vi "DAQ_SampleLoopSub.vi"(0 "DAQ_collectQueue":refnum<queue>, 1 "SampleSettings":T1={"samples per channel"=100, "SampleRate"=1000.0, "TansMaxLength"=500000.0, "ReadTimeOut"=10.0, "时钟源"=""}, 2 "AI_task":refnum<k21> caption="AITask", 3 "CntTask 1":refnum<k21> caption="CntTask1", 4 "CntTask 2":refnum<k21> caption="CntTask2", 6 "ClearCnt":bool, 8 "sensor_arrtribute":cluster{"Scale":dbl, "Offset":dbl}[](array[cluster])) -> (15 "RealTimeValue":dbl[](array[numeric]))   [LabVIEW 2020, in "DAQ.lvlib" / "NI_DAQ.lvclass"]
uses:
  NI_DAQ.lvclass
  DAQ_Base_class/protected/SampleSettings.ctl
  <vilib>/DAQmx/read.llb/DAQmx Read (Counter 1D DBL 1Chan NSamp).vi
  <vilib>/DAQmx/read.llb/DAQmx Read (Analog 2D DBL NChan NSamp).vi
  <vilib>/DAQmx/miscellaneous.llb/DAQmx Fill In Error Info.vi
  DAQ_Base_class/DAQ_Base.lvclass
panel:
  out "error out":errorcluster
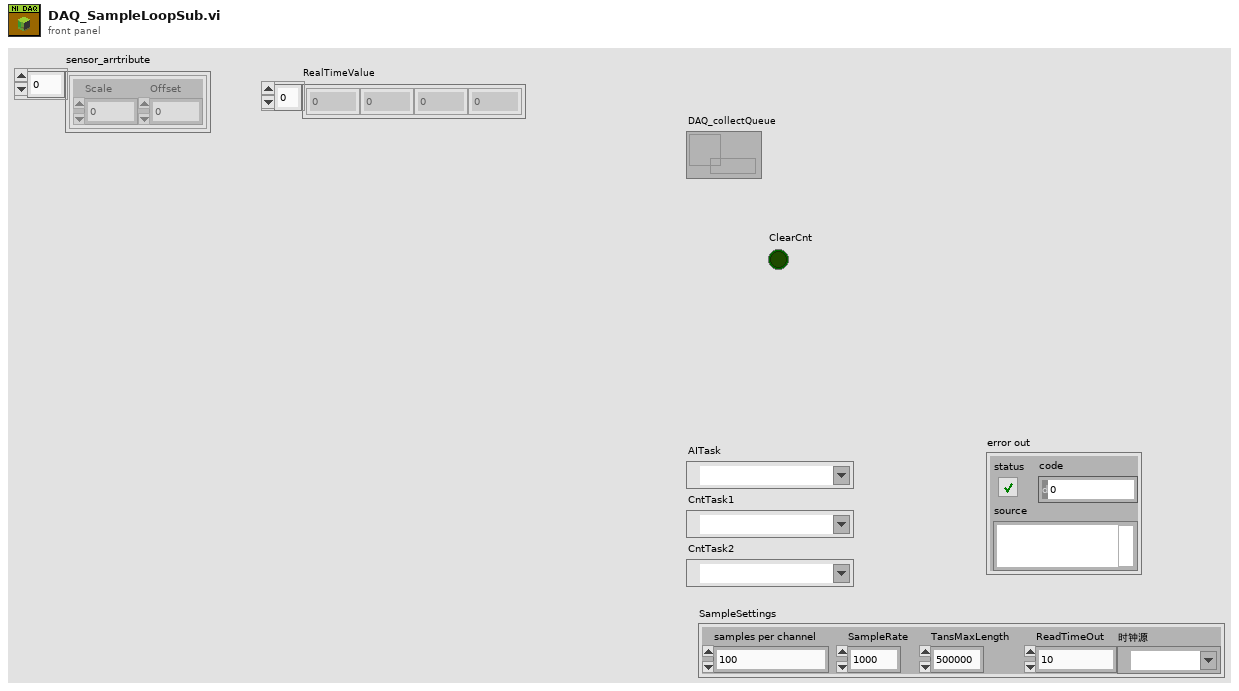
[diagram p1: front panel]
types:
  T1 = typedef "DAQ.lvlib/DAQ_Base.lvclass/SampleSettings.ctl" = cluster{"samples per channel":i32, "SampleRate":dbl, "TansMaxLength":dbl, "ReadTimeOut":dbl, "时钟源":tag}
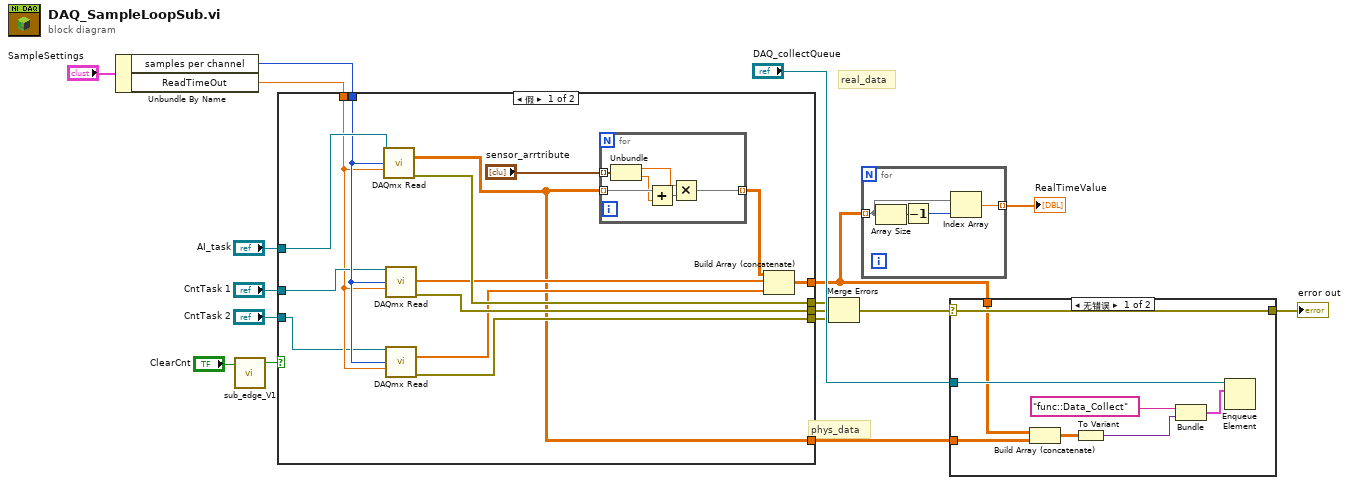
[diagram p0: block diagram]
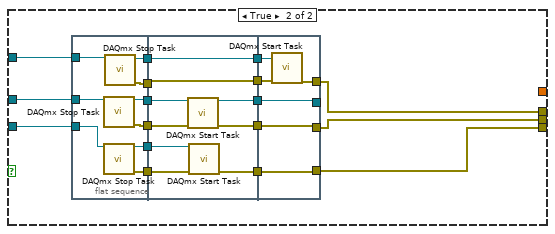
[diagram p2: hidden frame]
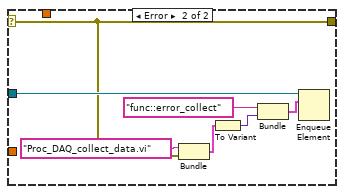
[diagram p3: hidden frame]
diagram:
  # "phys_data"
  # "real_data"
  n1 = Unbundle By Name("SampleSettings") -> ("samples per channel"=w9:i32, "ReadTimeOut"=w3:dbl)
  n2 = call "sub_edge_V1.vi"("signal_in"="ClearCnt") -> ("raise_edge"=w7:bool)  [unwired: 8 in, 2 out]
  n3 = case shown="假" w7 {
    tunnel: [w31 w46] -> w15
    tunnel: [w30 w45] -> w14
    tunnel: [w29 w44] -> w13
    tunnel: "AI_task" -> [w26 w43]
    tunnel: w9 -> [w25 _]
    tunnel: "CntTask 1" -> [w24 w42]
    tunnel: "CntTask 2" -> [w22 w41]
    tunnel: [w18 _] -> w1
    tunnel: [w20 _] -> w4
    tunnel: w3 -> [w23 _]
    frame False {
      n4 = call-poly <vilib>:"DAQmx Read.vi"("task/channels in"=w26, "number of samples per channel"=w25, "timeout"=w23) -> ("data"=w20:dbl[][], "error out"=w31:errorcluster)  [unwired: 10 in, 1 out]
      n5 = call-poly <vilib>:"DAQmx Read.vi"("task/channels in"=w24, "number of samples per channel"=w25, "timeout"=w23) -> ("data"=w27:dbl[], "error out"=w30:errorcluster)  [unwired: 10 in, 1 out]
      n6 = call-poly <vilib>:"DAQmx Read.vi"("task/channels in"=w22, "number of samples per channel"=w25, "timeout"=w23) -> ("data"=w28:dbl[], "error out"=w29:errorcluster)  [unwired: 10 in, 1 out]
      n7 = for {
        tunnel: w20 -> [w36] mode=indexing
        tunnel: "sensor_arrtribute" -> [w37] mode=indexing
        tunnel: [w32] -> w19 mode=indexing
        n8 = Unbundle(w37) -> ("Scale"=w35:dbl, "Offset"=w33:dbl)
        n9 = Add(x=w36, y=w33) -> (x+y=w34:dbl[])
        n10 = Multiply(x=w35, y=w34) -> (x*y=w32:dbl[])
      }
      n11 = Build Array (concatenate)(w19, w27, w28) -> (w18:dbl[][])
    }
    frame True {
      n12 = flat-sequence {
        tunnel: [w61] -> w54
        tunnel: [w60] -> w53
        tunnel: [w63] -> w52
        tunnel: [w62] -> w51
        tunnel: [w59] -> w50
        tunnel: [w58] -> w49
        tunnel: w43 -> [w57]
        tunnel: w42 -> [w56]
        tunnel: w41 -> [w55]
        tunnel: [w72] -> w48
        tunnel: [w71] -> w47
        tunnel: w54 -> [w69]
        tunnel: w53 -> [w70]
        tunnel: w52 -> [w66]
        tunnel: w51 -> [w65]
        tunnel: w50 -> [w67]
        tunnel: w49 -> [w68]
        tunnel: [w66] -> w40
        tunnel: [w65] -> w39
        tunnel: [w64] -> w38
        tunnel: [w73] -> w44
        tunnel: [w78] -> _
        tunnel: [w77] -> w45
        tunnel: [w74] -> w46
        tunnel: w48 -> [w78]
        tunnel: w47 -> [w77]
        tunnel: w40 -> [w76]
        tunnel: w39 -> [w75]
        tunnel: w38 -> [w73]
        frame #0 {
          n13 = call <vilib>:"DAQmx Stop Task.vi"("task/channels in"=w56) -> ("task out"=w61:refnum<k21>, "error out"=w60:errorcluster)  [unwired: 13 in]
          n14 = call <vilib>:"DAQmx Stop Task.vi"("task/channels in"=w55) -> ("task out"=w58:refnum<k21>, "error out"=w59:errorcluster)  [unwired: 13 in]
          n15 = call <vilib>:"DAQmx Stop Task.vi"("task/channels in"=w57) -> ("task out"=w63:refnum<k21>, "error out"=w62:errorcluster)  [unwired: 13 in]
        }
        frame #1 {
          n16 = call <vilib>:"DAQmx Start Task.vi"("task/channels in"=w69, "error in"=w70) -> ("task out"=w72:refnum<k21>, "error out"=w71:errorcluster)  [unwired: 12 in]
          n17 = call <vilib>:"DAQmx Start Task.vi"("task/channels in"=w68, "error in"=w67) -> ("error out"=w64:errorcluster)  [unwired: 12 in, 1 out]
        }
        frame #2 {
          n18 = call <vilib>:"DAQmx Start Task.vi"("task/channels in"=w76, "error in"=w75) -> ("error out"=w74:errorcluster)  [unwired: 12 in, 1 out]
        }
      }
    }
  }
  n19 = Merge Errors(w15, w14, w13) -> (w12:errorcluster)
  n20 = for {
    tunnel: w1 -> [w82] mode=indexing
    tunnel: [w81] -> w2 mode=indexing
    n21 = Array Size(array=w82) -> (size(s)=w80:i32)
    n22 = Decrement(x=w80) -> (x-1=w79:i32)
    n23 = Index Array(array=w82, index=w79) -> (element=w81:dbl)
  }
  "RealTimeValue" <- w2
  n24 = case shown="无错误" w12 {
    selector: w12 -> [w86 w91]
    tunnel: "DAQ_collectQueue" -> [w90 w97]
    tunnel: [w86 w91] -> w16
    tunnel: w1 -> [w85 _]
    tunnel: w4 -> [w84 _]
    frame No Error {
      n25 = Build Array (concatenate)(w85, w84) -> (w83:dbl[][])
      n26 = To Variant(anything=w83) -> (Variant=w87:variant)
      n27 = Bundle("func::Data_Collect", "Variant"=w87) -> (w88:cluster{string, "Variant":variant})  [unwired: 1 in]
      n28 = Enqueue Element(queue=w90, element=w88) -> ()  [unwired: 2 in, 3 out]
    }
    frame Error {
      n29 = Bundle("Proc_DAQ_collect_data.vi", "error IO"=w91) -> (w92:cluster{string, "error IO":errorcluster})  [unwired: 1 in]
      n30 = To Variant(anything=w92) -> (Variant=w94:variant)
      n31 = Bundle("func::error_collect", "Variant"=w94) -> (w95:cluster{string, "Variant":variant})  [unwired: 1 in]
      n32 = Enqueue Element(queue=w97, element=w95) -> ()  [unwired: 2 in, 3 out]
    }
  }
  "error out" <- w16
